vi "LDO_Update_Intellifaucet_Parameters.vi"(8 "error in (no error)":errorcluster, 9 "Valve % Open - Automatic Mode":dbl=15.0 min=15.0 max=100.0, 10 "Temp (°F) - Automatic Mode":dbl=32.0 min=32.0 max=203.0, 11 "Modbus Input":refnum<queue>) -> (0 "error out":errorcluster)   [LabVIEW 2020]
uses:
  Message Queue/Message Cluster.ctl
  Message Queue/Enqueue Message (Single).vi
  Message Queue/Message Queue.lvlib
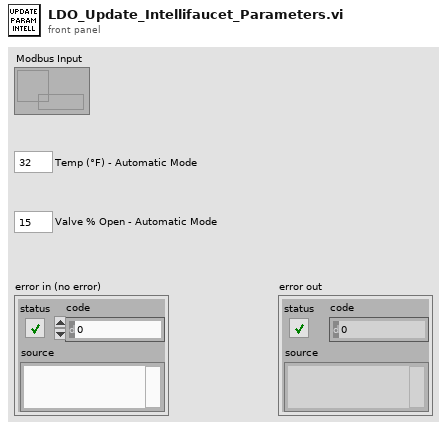
[diagram p1: front panel]
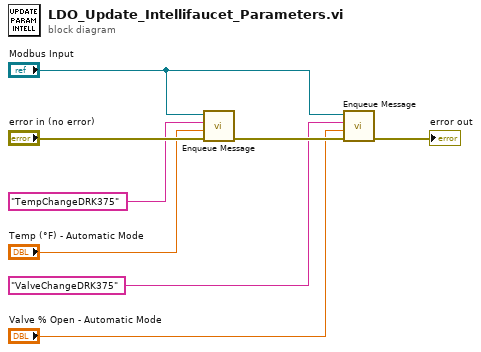
[diagram p0: block diagram]
diagram:
  n1 = call-poly "Enqueue Message.vi"("error in (no error)"="error in (no error)", "Message Data"="Temp (°F) - Automatic Mode", "Message"="TempChangeDRK375", "Message Queue"="Modbus Input") -> ("error out"=w6:errorcluster)  [unwired: 6 in, 1 out]
  n2 = call-poly "Enqueue Message.vi"("error in (no error)"=w6, "Message Data"="Valve % Open - Automatic Mode", "Message"="ValveChangeDRK375", "Message Queue"="Modbus Input") -> ("error out"=→"error out":errorcluster)  [unwired: 6 in, 1 out]
